vi "4.4.vi"() -> ()   [LabVIEW 2017]
panel:
  in  "use system alert? (T)":bool=TRUE caption="使用系统警报？(T)"
  in  "数值":dbl
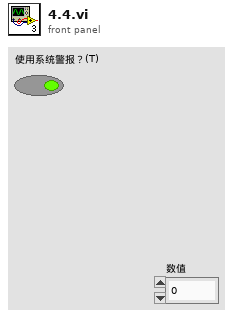
[diagram p1: front panel]
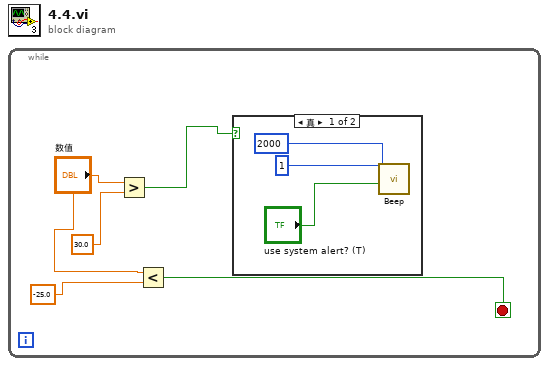
[diagram p0: block diagram]
diagram:
  n1 = while {
    stop <- w2 stop-if-true
    n2 = Greater?(x="数值", y=30.0 ("数值")) -> (0:w1:bool)
    n3 = Less?(x="数值", y=-25.0 ("数值 2")) -> (x < y?=w2:bool)
    n4 = case shown="真" w1 {
      frame True {
        n5 = call <vilib>:"Beep.vi"("use system alert? (T)"="use system alert? (T)", "duration (msec)"=u32 1, "frequency (Hz)"=u32 2000) -> ()  [unwired: 9 in]
      }
      frame False {
      }
    }
  }
